vi "Set Strings from Ref.vi"(8 "error in (no error)":errorcluster, 9 "Language Index (0)":i32, 10 "GObj Refnum":refnum<vi>, 11 "ArrayConstant in":refnum<class "ArrayControl.lvclass">) -> (0 "error out":errorcluster, 3 "ArrayConstant out":refnum<class "ArrayControl.lvclass">)   [LabVIEW 2013, in "SET Project Data.lvlib" / "ArrayControl.lvclass"]
uses:
  ArrayControl.lvclass
  Control/Control.lvclass
  SET Project Data.lvlib
  GObject/GObject.lvclass
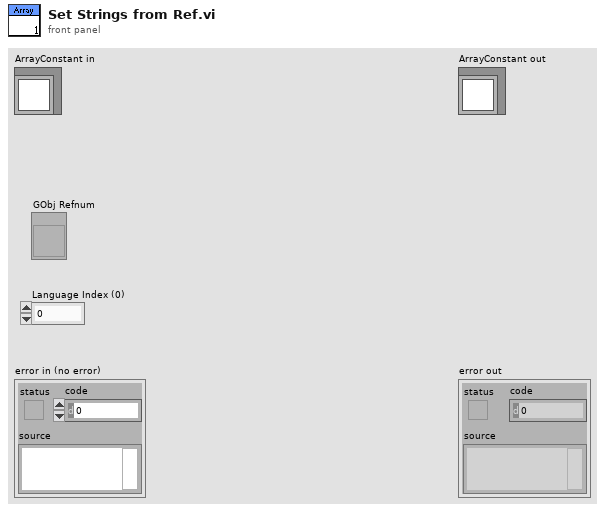
[diagram p1: front panel]
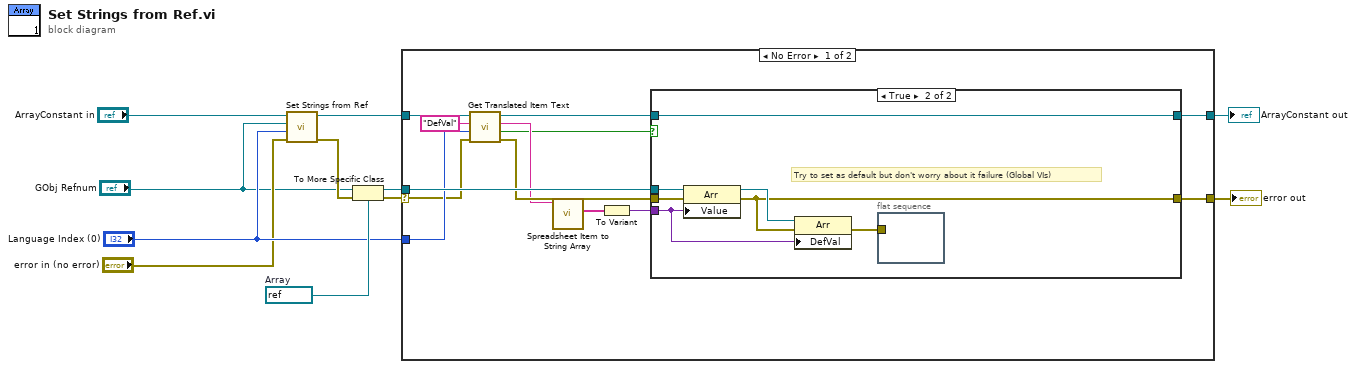
[diagram p0: block diagram]
diagram:
  w8 = refnum<vi> refnum  # Array
  n1 = call-parent "Set Strings from Ref.vi"("error in (no error)"="error in (no error)", "Language Index (0)"="Language Index (0)", "GObj Refnum"="GObj Refnum", "Control in"="ArrayConstant in") -> ("error out"=w11:errorcluster, "Control out"=w7:refnum<class "ArrayControl.lvclass">)  [unwired: 6 in]
  n2 = To More Specific Class(target class=w8, reference="GObj Refnum", error in=w11) -> (specific class reference=w9:refnum<vi>, error out=w10:errorcluster)
  n3 = case shown="No Error" w10 {
    selector: w10 -> [w21 w34]
    tunnel: w9 -> [w24 _]
    tunnel: w7 -> [w23 w35]
    tunnel: [w12 w35] -> w1
    tunnel: "Language Index (0)" -> [w22 _]
    tunnel: [w20 w34] -> w2
    frame No Error {
      n4 = call "Get Translated Item Text.vi"("error in (no error)"=w21, "LangIndex (0)"=w22, "ItemName"="DefVal", "GObject in"=w23) -> ("error out"=w18:errorcluster, "Found?"=w14:bool, "Translated Text (ASCII)"=w17:string, "GObject out"=w13:refnum<class "ArrayControl.lvclass">)  [unwired: 4 in]
      n5 = call "Spreadsheet Item to String Array.vi"("Spreadsheet Item (ASCII)"=w17) -> ("Strings [] (ASCII)"=w16:string[])  [unwired: 10 in]
      n6 = To Variant(anything=w16) -> (Variant=w15:variant)
      n7 = case shown="True" w14 {
        tunnel: w24 -> [_ w33]
        tunnel: w15 -> [_ w31]
        tunnel: w18 -> [w26 w29]
        tunnel: [w26 w28] -> w20
        tunnel: w13 -> [w25 w30]
        tunnel: [w25 w30] -> w12
        frame False {
        }
        frame True {
          # "Try to set as default but don't worry about it failure (Global VIs)"
          n8 = property class="Arr"(reference=w33, error in=w29, "Value"=w31) -> (reference out=w32:refnum<vi>, error out=w28:errorcluster)
          n9 = property class="Arr"(reference=w32, error in=w28, "DefVal"=w31) -> (error out=w27:errorcluster)  [unwired: 1 out]
          n10 = flat-sequence {
            tunnel: w27 -> [_]
            frame #0 {
            }
          }
        }
      }
    }
    frame Error {
    }
  }
  "error out" <- w2
  "ArrayConstant out" <- w1
